vi "ConfigureAnalogOutputs.vi"(0 "axis in":cluster{"keyHandle":u32, "nodeId":u16}={"keyHandle"=0, "nodeId"=1}, 9 "analog output configuration":T1={"analogOutputNumber"=1, "configuration"=0} {"configuration" items=["general purpose A", "general purpose B"]}, 11 "error in (no error)":errorcluster) -> (4 "axis out":cluster{"keyHandle":u32, "nodeId":u16}={"keyHandle"=0, "nodeId"=1}, 15 "error out":errorcluster)   [LabVIEW 2019, in "maxonEPOS.lvlib"]
doc: "<B>ConfigureAnalogInputs</B> writes the configuration parameters for an analog input to the device."
uses:
  Examples/maxonEPOS.lvlib
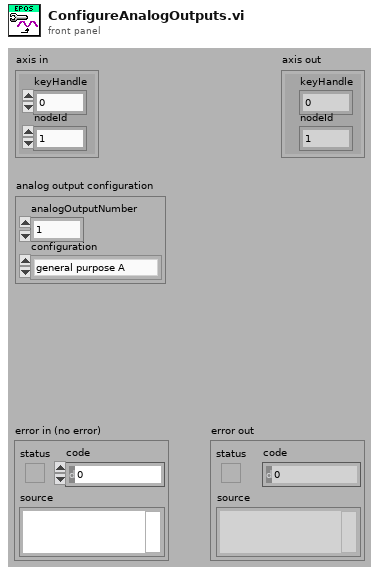
[diagram p1: front panel]
types:
  T1 = cluster{"analogOutputNumber":u16, "configuration":u16}
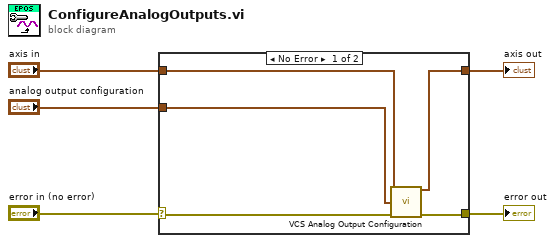
[diagram p0: block diagram]
diagram:
  n1 = case shown="No Error" "error in (no error)" {
    selector: "error in (no error)" -> [w7 w12]
    tunnel: [w10 w12] -> w4
    tunnel: [w9 w11] -> w3
    tunnel: "axis in" -> [w6 w11]
    tunnel: "analog output configuration" -> [w8 _]
    frame No Error {
      n2 = call "VCS Analog Output Configuration.vi"("axis in"=w6, "configuration"=w8, "error in (no error)"=w7) -> ("axis out"=w9:cluster{"keyHandle":u32, "nodeId":u16}, "error out"=w10:errorcluster)  [unwired: 11 in]
    }
    frame Error {
    }
  }
  "error out" <- w4
  "axis out" <- w3
